vi "Module Loop.vi"(8 "error in (no error)":errorcluster, 11 "Event Viewer Module in":refnum<class "Event Viewer Module.lvclass">) -> (0 "error out":errorcluster, 3 "Event Viewer Module out":refnum<class "Event Viewer Module.lvclass">)   [LabVIEW 2020, in "VolatusGUI.lvlib" / "Event Viewer Module.lvclass"]
uses:
  Event Viewer Module.lvclass
  C:/dev/lv20CE/relink/lv-volatus/Volatus/Module/Module.lvclass
  Event Element.ctl
  Volatus/Module/Module.lvclass/Module.ctl
  Volatus/MessageQ/MessageQ.lvclass/MessageQ.ctl
  Event Viewer Module.lvclass/Event Viewer Module.ctl
  Volatus/Module/Module.lvclass
  Event Filters.ctl
  Volatus/Events Summary Value/Events Summary Value.lvclass
  Volatus/PathValue/PathValue.lvclass
  Volatus/PathValue/PathValue.lvclass/PathValue.ctl
  Volatus/Event.ctl
  Volatus/Event Level.ctl
  <vilib>/AdvancedString/Delimited String to 1D String Array.vi
  <vilib>/dlg_ctls.llb/Space Constant.vi
  <vilib>/Utility/error.llb/Error Cluster From Error Code.vi
  Volatus/MessageQ/MessageQ.lvclass
  GUI Helper/GUI Helper.lvclass
  Volatus/Volatus.lvlib
  GUI Info.ctl
  VolatusGUI.lvlib
panel:
  in  "Source Filter":string(combo) caption="Source Filter..."
  in  "Clear Events":bool
  in  "Show Log":bool
  in  "Reset Filters":bool
  in  "Error":bool=TRUE
  in  "Warning":bool=TRUE
  in  "Info":bool=TRUE
  in  "Debug":bool
  in  "Text Filter":string caption="Text Filter..."
  out "# Debug":i32
  out "# Warning":i32
  out "# Info":i32
  out "# Error":i32
  out "Events":T1[](array[typedef])
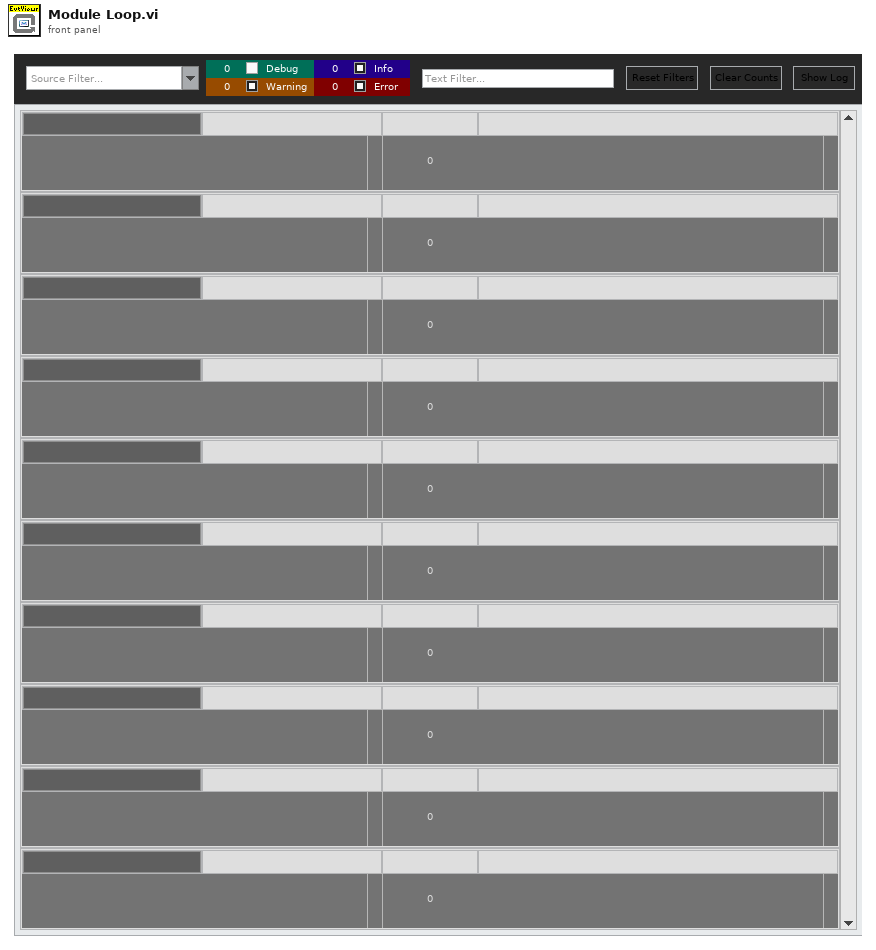
[diagram p1: front panel]
types:
  T1 = typedef "VolatusGUI.lvlib/Event Viewer Module.lvclass/Event Element.ctl" = cluster{"Node":string, "Node Color":u32, "Timestamp":string, "TS Color":u32, "Level":string, "Level Color":u32, "Context":string, "Context Color":u32, "Message":string, "Error Code":i32, "Error Source":string}
  T2 = enum32{"Invalid", "Standard", "Closed", "Hidden", "Minimized", "Maximized"}
  T3 = typedef "VolatusGUI.lvlib/Event Viewer Module.lvclass/Event Filters.ctl" = cluster{"Source":string, "Text":string, "Debug":bool, "Info":bool, "Warning":bool, "Error":bool}
  T4 = typedef "VolatusGUI.lvlib/GUI Info.ctl" = cluster{"Color":u32, "Name":string}
  T5 = typedef "Volatus.lvlib/Event.ctl" = cluster{"Time Stamp":timestamp, "Event Level":T6, "Context":string, "Message":string, "Error":errorcluster, "Node":string}
  T6 = typedef "Volatus.lvlib/Event Level.ctl" = enum16{"Debug", "Info", "Warning", "Error"}
  T7 = typedef "Volatus.lvlib/Events Summary.ctl" = cluster{"# Debug":i32, "# Info":i32, "# Warning":i32, "# Error":i32}
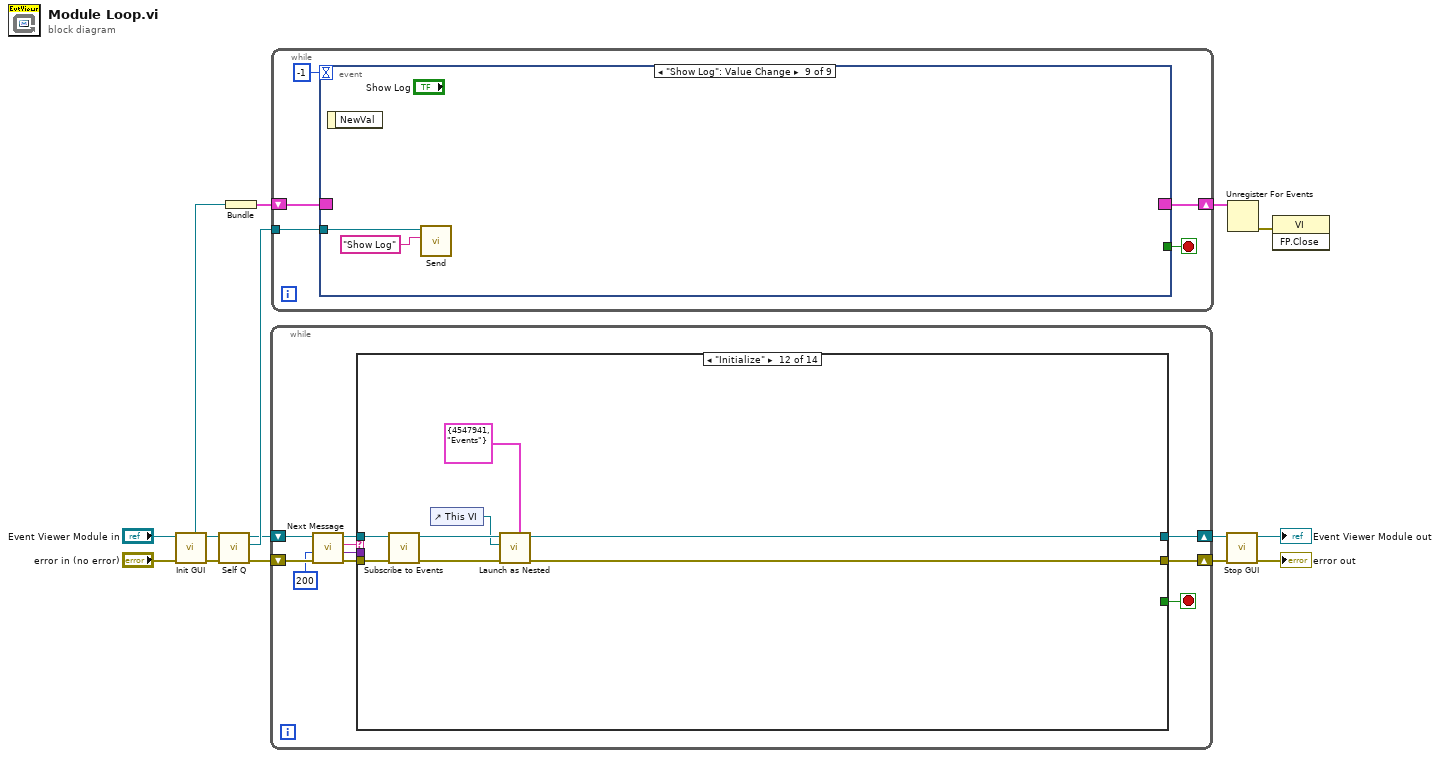
[diagram p0: block diagram]
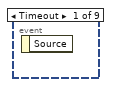
[diagram p2: hidden frame]
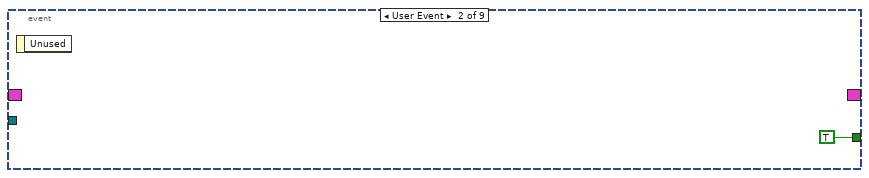
[diagram p3: hidden frame]
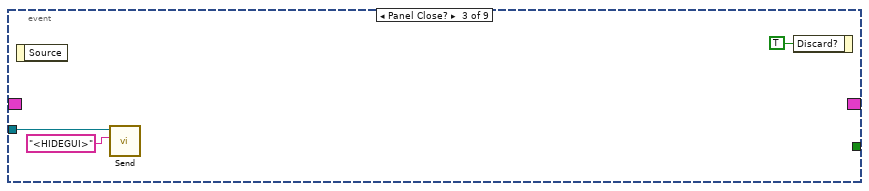
[diagram p4: hidden frame]
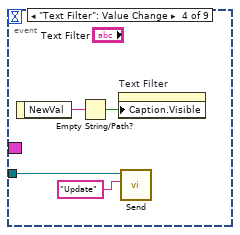
[diagram p5: hidden frame]
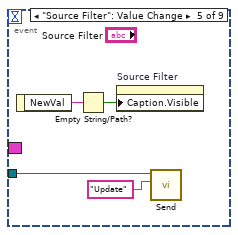
[diagram p6: hidden frame]
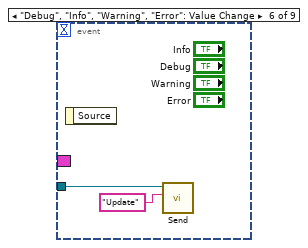
[diagram p7: hidden frame]
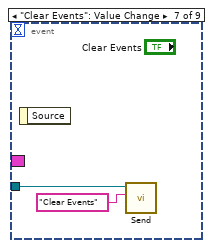
[diagram p8: hidden frame]
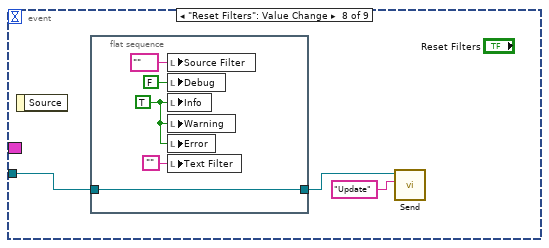
[diagram p9: hidden frame]
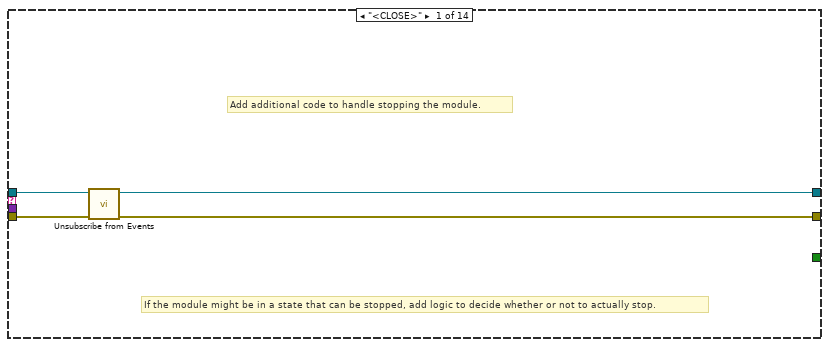
[diagram p10: hidden frame]
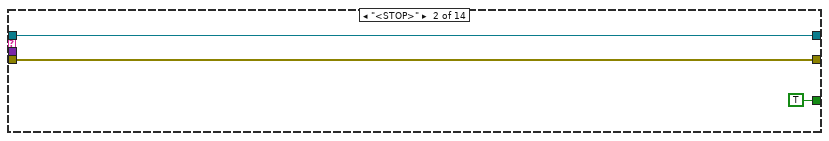
[diagram p11: hidden frame]
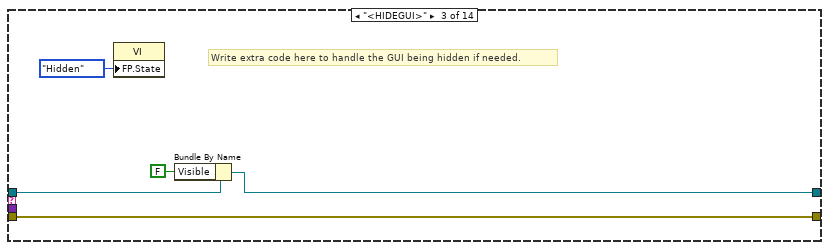
[diagram p12: hidden frame]
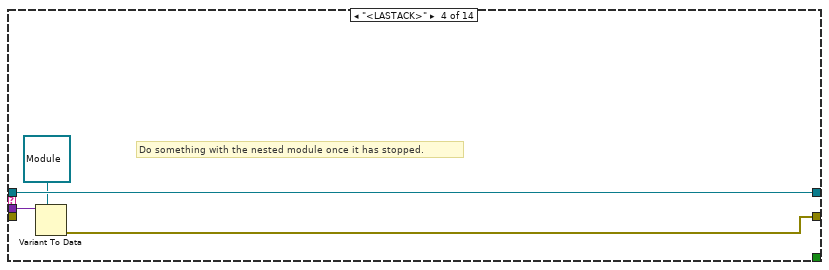
[diagram p13: hidden frame]
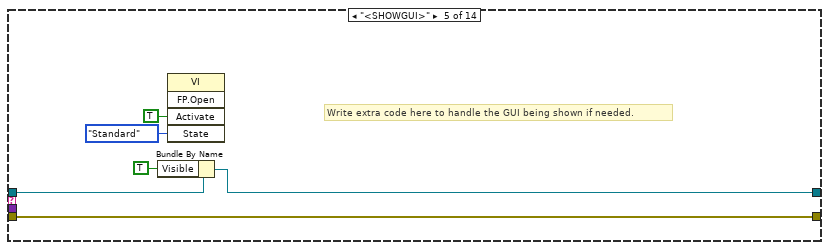
[diagram p14: hidden frame]
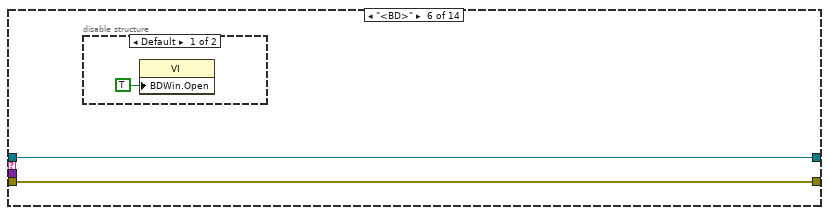
[diagram p15: hidden frame]
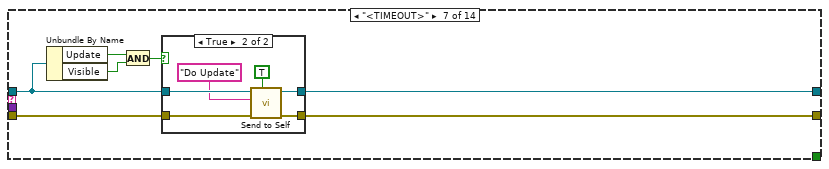
[diagram p17: hidden frame]
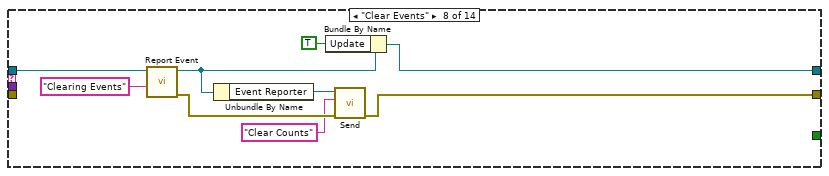
[diagram p19: hidden frame]
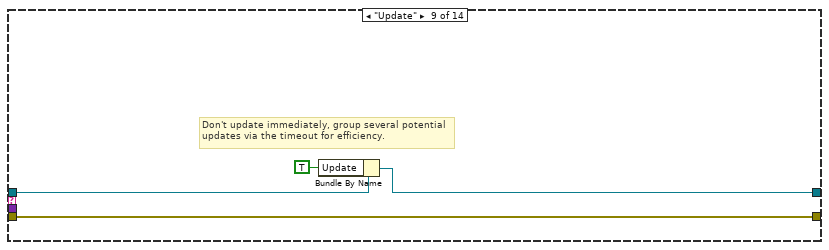
[diagram p20: hidden frame]
diagram:
  n1 = call "Init GUI.vi"("Module in"="Event Viewer Module in") -> ("Module out"=w7:refnum<class "Event Viewer Module.lvclass">, "Event Reg"=w12:refnum<event-registration>)  [unwired: 9 in]
  n2 = call "Self Q.vi"("Module in"=w7) -> ("Self Q"=w6:refnum<class "MessageQ.lvclass">, "Module out"=w5:refnum<class "Event Viewer Module.lvclass">)  [unwired: 9 in]
  n3 = Bundle("Event Reg"=w12) -> (w8:cluster{"Event Reg":refnum<event-registration>})  [unwired: 1 in]
  n4 = while {
    shift-right: [w18] -> w10
    shift-left: w5 -> [w23]
    shift-right: [w17] -> w11
    shift-left: "error in (no error)" -> [w22]
    stop <- w16 stop-if-true
    n5 = call "Next Message.vi"("error in (no error)"=w22, "Timeout ms (-1)"=200, "Module in"=w23) -> ("error out"=w21:errorcluster, "Data"=w15:variant, "ID"=w20:string, "Module out"=w19:refnum<class "Event Viewer Module.lvclass">)  [unwired: 5 in]
    n6 = case shown="\"Initialize\"" w20 {
      tunnel: w21 -> [w27 w29 w34 _ w44 w46 w55 _ w75 w105 _ w121 _ w137]
      tunnel: w19 -> [w25 w30 w35 w39 w45 w47 w52 w71 w76 w88 w113 w119 w130 w135]
      tunnel: [w24 w30 w32 w39 w41 w47 w53 w67 w74 w104 w113 w116 w125 w134] -> w18
      tunnel: [w26 w29 w34 w36 w44 w46 w54 w68 w75 w105 w106 w118 w126 w136] -> w17
      tunnel: [_ TRUE _ _ _ _ _ _ _ _ _ _ _ _] -> w16
      tunnel: w15 -> [_ _ _ w38 _ _ _ _ _ _ _ _ w132 _]
      frame "<CLOSE>" {
        # "If the module might be in a state that can be stopped, add logic to decide whether or not to actually stop."
        # "Add additional code to handle stopping the module."
        n7 = call "Unsubscribe from Events.vi"("error in (no error)"=w27, "Event Viewer Module in"=w25) -> ("error out"=w26:errorcluster, "Event Viewer Module out"=w24:refnum<class "Event Viewer Module.lvclass">)  [unwired: 8 in]
      }
      frame "<STOP>" {
      }
      frame "<HIDEGUI>" {
        # "Write extra code here to handle the GUI being hidden if needed."
        n8 = property class="VI"("FP.State"=T2."Hidden" ("Front Panel Window:State")) -> ()  [unwired: 2 in, 2 out]
        n9 = Bundle By Name(cluster=w35, "Visible"=FALSE) -> (w32:refnum<class "Event Viewer Module.lvclass">)
      }
      frame "<LASTACK>" {
        # "Do something with the nested module once it has stopped."
        n10 = Variant To Data(type=refnum<class "Module.lvclass"> refnum ("Volatus:Module"), Variant=w38) -> (error out=w36:errorcluster)  [unwired: 1 in, 1 out]
      }
      frame "<SHOWGUI>" {
        # "Write extra code here to handle the GUI being shown if needed."
        n11 = Bundle By Name(cluster=w45, "Visible"=TRUE) -> (w41:refnum<class "Event Viewer Module.lvclass">)
        n12 = invoke class="VI" method="FP.Open"("Activate"=TRUE ("Activate?"), "State"=T2."Standard") -> ()  [unwired: 3 in, 5 out]
      }
      frame "<BD>" {
        n13 = disable-structure shown="Default" {
          frame condition #0 (active) {
            n14 = property class="VI"("BDWin.Open"=TRUE ("Block Diagram Window:Open")) -> ()  [unwired: 2 in, 2 out]
          }
          frame condition #1 {
          }
        }
      }
      frame "<TIMEOUT>" {
        n15 = Unbundle By Name(w52) -> ("Update"=w51:bool, "Visible"=w50:bool)
        n16 = And(x=w51, y=w50) -> (x .and. y?=w49:bool)
        n17 = case shown="False" w49 {
          tunnel: w55 -> [w56 w63]
          tunnel: [w56 w62] -> w54
          tunnel: [w57 w61] -> w53
          tunnel: w52 -> [w57 w60]
          frame False {
          }
          frame True {
            n18 = call "Send to Self.vi"("High Priority (F)"=TRUE, "error in (no error)"=w63, "Message ID"="Do Update", "Module in"=w60) -> ("error out"=w62:errorcluster, "Module out"=w61:refnum<class "Event Viewer Module.lvclass">)  [unwired: 6 in]
          }
        }
      }
      frame "Clear Events" {
        n19 = call "Report Event.vi"("Message"="Clearing Events", "Module in"=w71) -> ("error out"=w72:errorcluster, "Module out"=w65:refnum<class "Event Viewer Module.lvclass">)  [unwired: 8 in]
        n20 = Unbundle By Name(w65) -> ("Event Reporter"=w70:refnum<class "MessageQ.lvclass">)
        n21 = Bundle By Name(cluster=w65, "Update"=TRUE) -> (w67:refnum<class "Event Viewer Module.lvclass">)
        n22 = call "Send.vi"("error in (no error)"=w72, "ID"="Clear Counts", "MessageQ in"=w70) -> ("error out"=w68:errorcluster)  [unwired: 7 in, 1 out]
      }
      frame "Update" {
        # "Don't update immediately, group several potential updates via the timeout for efficiency."
        n23 = Bundle By Name(cluster=w76, "Update"=TRUE) -> (w74:refnum<class "Event Viewer Module.lvclass">)
      }
      frame "Do Update" {
        n24 = local read "Source Filter"() -> (w90:string)
        n25 = Unbundle By Name(w88) -> ("Events"=w102:refnum<queue>)
        n26 = local read "Text Filter"() -> (w91:string)
        n27 = local read "Warning"() -> (w94:bool)
        n28 = local read "Debug"() -> (w92:bool)
        n29 = local read "Error"() -> (w95:bool)
        n30 = local read "Info"() -> (w93:bool)
        n31 = Get Queue Status(queue=w102, return elements? (F)=TRUE) -> (elements=w100:T1[])  [unwired: 1 in, 7 out]
        n32 = Bundle By Name(cluster=T3 {"Source"="", "Text"="", "Debug"=FALSE, "Info"=FALSE, "Warning"=FALSE, "Error"=FALSE} ("Event Filters"), "Source"=w90, "Text"=w91, "Debug"=w92, "Info"=w93, "Warning"=w94, "Error"=w95) -> (w89:T3)
        n33 = call "Source Names.vi"("Events in"=w100) -> ("Sources"=w97:string[], "Events"=w99:T1[])  [unwired: 5 in]
        n34 = call "Filter Events.vi"("Events"=w99, "Event Filters"=w89) -> ("Filtered Events"=w98:T1[])  [unwired: 5 in]
        n35 = Reverse 1D Array(array=w98) -> (reversed array=→"Events":T1[])
        n36 = property on="Source Filter" class="CmbBox"("Strings[]"=w97) -> ()  [unwired: 2 in, 2 out]
        n37 = Unbundle By Name(w88) -> ("Event Reporter"=w87:refnum<class "MessageQ.lvclass">)
        n38 = call "Request.vi"("Response Type (None)"=refnum<class "Events Summary Value.lvclass"> refnum ("Volatus:Events Summary Value.lvclass"), "Timeout ms (1000)"=100, "ID"="Request Event Summary", "MessageQ in"=w87) -> ("Response"=w84:refnum<class "Events Summary Value.lvclass">)  [unwired: 5 in, 2 out]
        n39 = call "Read.vi"("Events Summary Value in"=w84) -> ("Events Summary"=w82:T7)  [unwired: 10 in]
        n40 = Unbundle By Name(w82) -> ("# Debug"=→"# Debug":i32, "# Info"=→"# Info":i32, "# Warning"=→"# Warning":i32, "# Error"=→"# Error":i32)
        n41 = Bundle By Name(cluster=w88, "Update"=FALSE) -> (w104:refnum<class "Event Viewer Module.lvclass">)
      }
      frame "Show Log" {
        # "Event Reporter knows where the log is saved on disk."
        n42 = Unbundle By Name(w113) -> ("Event Reporter"=w112:refnum<class "MessageQ.lvclass">)
        n43 = call "Request.vi"("Response Type (None)"=refnum<class "PathValue.lvclass"> refnum ("Volatus:PathValue.lvclass"), "ID"="Request Log Path", "MessageQ in"=w112) -> ("error out"=w108:errorcluster, "Response"=w110:refnum<class "PathValue.lvclass">)  [unwired: 6 in, 1 out]
        n44 = call "Read.vi"("PathValue in"=w110) -> ("Path"=w107:path)  [unwired: 10 in]
        n45 = call <vilib>:"Show in File System.vi"("error in (no error)"=w108, "file or directory path"=w107) -> ("error out"=w106:errorcluster)  [unwired: 9 in]
      }
      frame "Initialize" {
        n46 = call "Subscribe to Events.vi"("error in (no error)"=w121, "Event Viewer Module in"=w119) -> ("error out"=w120:errorcluster, "Event Viewer Module out"=w117:refnum<class "Event Viewer Module.lvclass">)  [unwired: 8 in]
        n47 = control-ref of="This VI"() -> (w115:refnum<vi>)
        n48 = call "Launch as Nested.vi"("GUI Info (Default)"=T4 {"Color"=4547941, "Name"="Events"}, "error in (no error)"=w120, "GUI"=w115, "Parent in"=w117) -> ("error out"=w118:errorcluster, "Parent"=w116:refnum<class "Event Viewer Module.lvclass">)  [unwired: 5 in, 1 out]
      }
      frame "New Event" {
        n49 = Variant To Data(type=T5 {"Time Stamp"=timestamp(0 s since 1904-01-01), "Event Level"=enum."Info", "Context"="", "Message"="", "Error"={"status"=FALSE, "code"=0, "source"=""}, "Node"=""} ("Event"), Variant=w132) -> (data=w131:T5, error out=w127:errorcluster)  [unwired: 1 in]
        n50 = call "Node Names.vi"("Module in"=w130) -> ("Node"=w122:string, "Module out"=w123:refnum<class "Event Viewer Module.lvclass">)  [unwired: 6 in, 3 out]
        n51 = call "Event to GUI Event.vi"("Event"=w131, "This Node"=w122) -> ("Event Element"=w128:T1)  [unwired: 5 in]
        n52 = Unbundle By Name(w123) -> ("Events"=w129:refnum<queue>)
        n53 = Bundle By Name(cluster=w123, "Update"=TRUE) -> (w125:refnum<class "Event Viewer Module.lvclass">)
        n54 = Enqueue Element(queue=w129, element=w128, error in (no error)=w127) -> (error out=w126:errorcluster)  [unwired: 1 in, 2 out]
      }
      frame Default {
        n55 = call "Report Unhandled Message ID.vi"("error in (no error)"=w137, "Module in"=w135) -> ("error out"=w136:errorcluster, "Module out"=w134:refnum<class "Event Viewer Module.lvclass">)  [unwired: 8 in]
      }
    }
  }
  n56 = while {
    tunnel: w6 -> [w142]
    shift-right: [w140] -> w9
    shift-left: w8 -> [w141]
    stop <- w139 stop-if-true
    n57 = event shown="[8] \"Show Log\": Value Change" {
      selector: w141 -> [_ _ _ _ _ _ _ _ _]
      dyn-events: [_ _ _ _ _ _ _ _ _] -> w140
      timeout: -1 -> [_ _ _ _ _ _ _ _ _]
      tunnel: w142 -> [_ _ w145 w148 w152 w156 w158 w160 w168]
      tunnel: [_ TRUE _ _ _ _ _ _ _] -> w139
      event Timeout {
        n58 = event-data() -> ()  [unwired: 1 in, 1 out]
      }
      event User Event {
        n59 = event-data() -> ()  [unwired: 1 in, 1 out]
      }
      event Panel Close? {
        n60 = event-data() -> ()  [unwired: 1 in, 1 out]
        n61 = call "Send.vi"("ID"="<HIDEGUI>", "MessageQ in"=w145) -> ()  [unwired: 8 in, 2 out]
        n62 = event-data("Discard?"=TRUE) -> ()  [unwired: 1 in, 1 out]
      }
      event "Text Filter": Value Change {
        n63 = event-data() -> ("NewVal"=w150:string)  [unwired: 1 in]
        n64 = Empty String/Path?(string/path=w150) -> (empty?=w149:bool)
        n65 = property on="Text Filter" class="Str"("Caption.Visible"=w149) -> ()  [unwired: 2 in, 2 out]
        n66 = call "Send.vi"("ID"="Update", "MessageQ in"=w148) -> ()  [unwired: 8 in, 2 out]
      }
      event "Source Filter": Value Change {
        n67 = event-data() -> ("NewVal"=w154:string)  [unwired: 1 in]
        n68 = Empty String/Path?(string/path=w154) -> (empty?=w153:bool)
        n69 = property on="Source Filter" class="CmbBox"("Caption.Visible"=w153) -> ()  [unwired: 2 in, 2 out]
        n70 = call "Send.vi"("ID"="Update", "MessageQ in"=w152) -> ()  [unwired: 8 in, 2 out]
      }
      event "Debug", "Info", "Warning", "Error": Value Change {
        n71 = event-data() -> ()  [unwired: 1 in, 1 out]
        n72 = call "Send.vi"("ID"="Update", "MessageQ in"=w156) -> ()  [unwired: 8 in, 2 out]
      }
      event "Clear Events": Value Change {
        n73 = event-data() -> ()  [unwired: 1 in, 1 out]
        n74 = call "Send.vi"("ID"="Clear Events", "MessageQ in"=w158) -> ()  [unwired: 8 in, 2 out]
      }
      event "Reset Filters": Value Change {
        n75 = event-data() -> ()  [unwired: 1 in, 1 out]
        n76 = flat-sequence {
          tunnel: w160 -> [w165]
          tunnel: [w165] -> w159
          frame #0 {
            w163 = TRUE ("Info")
            n77 = local write "Source Filter"("" ("Source Filter")) -> ()
            n78 = local write "Debug"(FALSE ("Debug")) -> ()
            n79 = local write "Info"(w163) -> ()
            n80 = local write "Warning"(w163) -> ()
            n81 = local write "Error"(w163) -> ()
            n82 = local write "Text Filter"("" ("Text Filter")) -> ()
          }
        }
        n83 = call "Send.vi"("ID"="Update", "MessageQ in"=w159) -> ()  [unwired: 8 in, 2 out]
      }
      event "Show Log": Value Change {
        n84 = event-data() -> ()  [unwired: 1 in, 1 out]
        n85 = call "Send.vi"("ID"="Show Log", "MessageQ in"=w168) -> ()  [unwired: 8 in, 2 out]
      }
    }
  }
  n86 = call "Stop GUI.vi"("error in (no error)"=w11, "Module in"=w10) -> ("error out"=→"error out":errorcluster, "Module out"=→"Event Viewer Module out":refnum<class "Event Viewer Module.lvclass">)  [unwired: 8 in]
  n87 = Unregister For Events(event registration refnum=w9) -> (error out=w13:errorcluster)  [unwired: 1 in]
  n88 = invoke class="VI" method="FP.Close"(error in=w13) -> ()  [unwired: 2 in, 3 out]
